vi "RTHost.vi"() -> ()   [LabVIEW 2013]
uses:
  <vilib>/Platform/TimedLoop/XDataNode/timing_clust.ctl
  <vilib>/Platform/TimedLoop/XDataNode/nitl_modes.ctl
  <vilib>/Platform/TimedLoop/XDataNode/wakeup.ctl
  <vilib>/FPGAPlugInAG/sbRIO-9632/niLvFpga_Open_sbRIO-9632.vi
  <vilib>/Utility/error.llb/Error Cluster From Error Code.vi
  <vilib>/rvi/errors/niLvFpgaAdjustHostInterfaceError.vi
  <vilib>/FPGAPlugInAG/sbRIO-9632/niLvFpga_Close_sbRIO-9632.vi
  <vilib>/rvi/interface/nirviOpenFPGA/nirviOpenFPGA.xnode
  FPGA Bitfiles/VMS15_FPGATarget_RTHost_BpHY6it1LyU.lvbitx
  <vilib>/rvi/interface/nirviReadWriteControl/nirviReadWriteControl.xnode
  <vilib>/Platform/TimedLoop/XDataNode/XDataNode.xnode
  <vilib>/rvi/interface/nirviCloseFPGA/nirviCloseFPGA.xnode
  NiFpgaLv.dll
  <vilib>/Platform/TimedLoop/XDataNode/XDNodeRunTimeDep.lvlib
panel:
  out "电池过温":bool
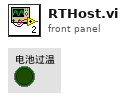
[diagram p1: front panel]
types:
  T1 = typedef "XDNodeRunTimeDep.lvlib/timing_clust.ctl" = cluster{"Expected End [f-1]":u64, "Actual End [f-1]":u64, "Finished Late? [f-1]":bool, "Expected End [i-1]":u64, "Actual End [i-1]":u64, "Finished Late? [i-1]":bool, "Expected Start [i]":u64, "Actual Start [i]":u64, "Expected Start [f]":u64, "Actual Start [f]":u64, "Source Name":string, "Structure Name":string, "Period":i64, "Deadline":i64, "Offset":i64, "Start":i64, "Priority":i32, "Timeout":i32, "Mode":T2, "Wakeup Reason":T3, "Error":errorcluster, "Source Type":string, "Secondary Source Type":string, "Global End Time":u64, "Global Start Time":u64, "Frame Duration":u64, "Iteration Duration":u64, "Assigned CPU":i32, "I/O Scan Engine Mode":u32}
  T2 = typedef "XDNodeRunTimeDep.lvlib/nitl_modes.ctl" = enum32{"No Change", "Process missed periods, maintain original phase", "Discard missed periods, maintain original phase", "Process missed periods, ignore original phase", "Discard missed periods, ignore original phase"}
  T3 = typedef "XDNodeRunTimeDep.lvlib/wakeup.ctl" = enum32{"Normal", "Aborted", "Asynchronous wakeup", "Timing source error", "Timed loop error", "Timeout"}
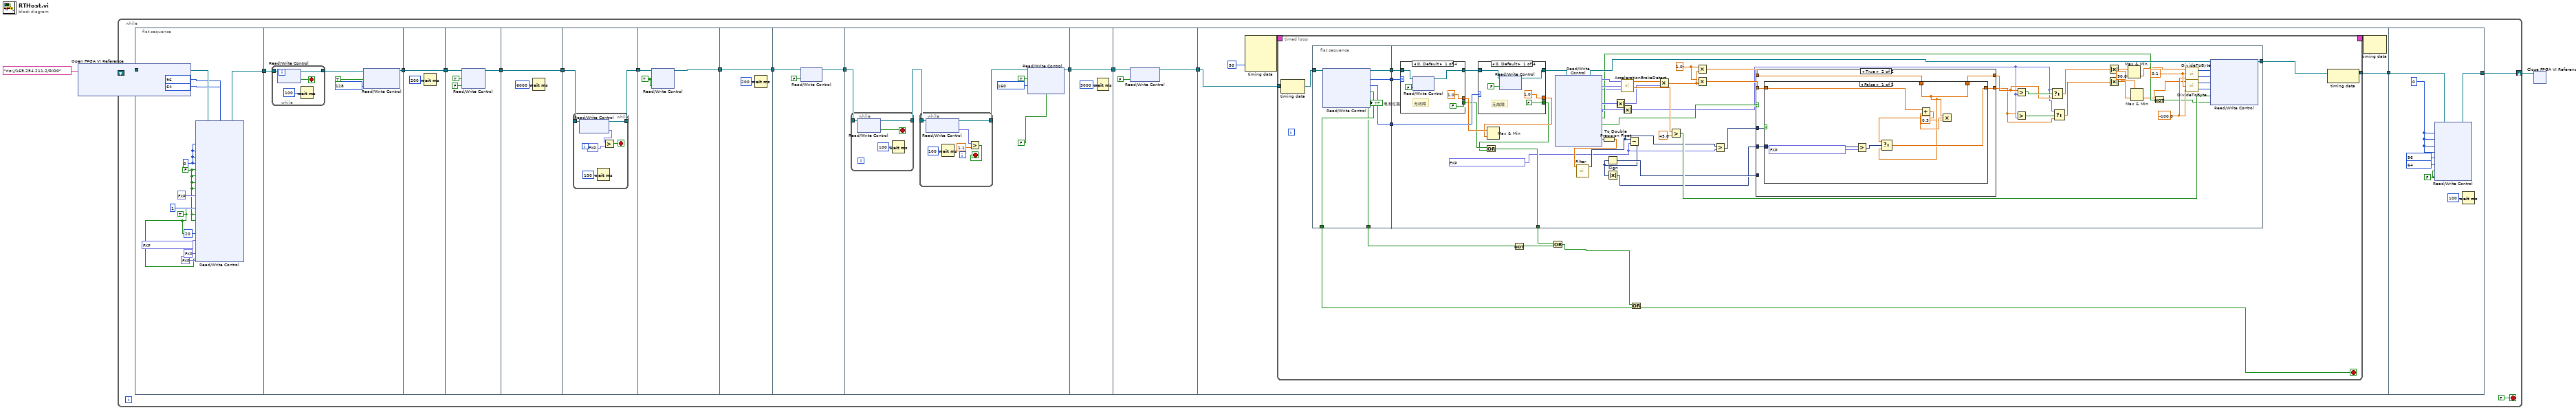
[diagram p0: block diagram]
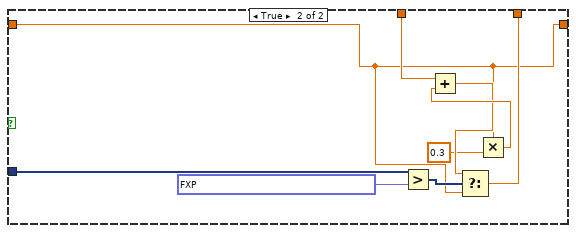
[diagram p3: hidden frame]
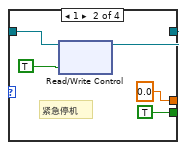
[diagram p4: hidden frame]
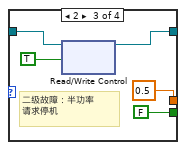
[diagram p5: hidden frame]
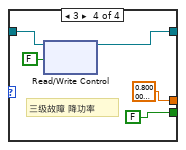
[diagram p6: hidden frame]
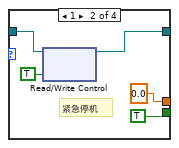
[diagram p7: hidden frame]
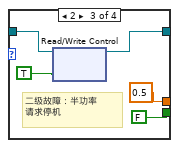
[diagram p8: hidden frame]
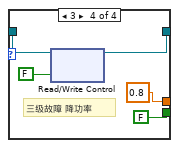
[diagram p9: hidden frame]
diagram:
  n1 = xnode "Open FPGA VI Reference"("resource name"=tag "rio://169.254.211.2/RIO0") -> ("FPGA VI Reference Out"=w1:refnum<k20>)  [unwired: 1 in, 1 out]
  n2 = while {
    shift-right: [w4] -> w2
    shift-left: w1 -> [w19]
    stop <- FALSE stop-if-true
    n3 = flat-sequence {
      tunnel: w19 -> [w29]
      tunnel: [w28] -> w18
      tunnel: w18 -> [w34]
      tunnel: [w33] -> w17
      tunnel: w17 -> [w43]
      tunnel: [w43] -> w16
      tunnel: w16 -> [w46]
      tunnel: [w45] -> w15
      tunnel: w15 -> [w49]
      tunnel: [w49] -> w10
      tunnel: [w51] -> w14
      tunnel: w10 -> [w50]
      tunnel: w14 -> [w60]
      tunnel: [w59] -> w7
      tunnel: w7 -> [w62]
      tunnel: [w62] -> w6
      tunnel: w6 -> [w65]
      tunnel: [w64] -> w5
      tunnel: w5 -> [w72]
      tunnel: [w67] -> w13
      tunnel: w13 -> [w84]
      tunnel: [w84] -> w9
      tunnel: [w86] -> w12
      tunnel: w9 -> [w87]
      tunnel: w12 -> [w90]
      tunnel: [w89] -> w11
      tunnel: w11 -> [w243]
      tunnel: [w238] -> w4
      frame #0 {
        w20 = TRUE ("AMS")
        w31 = u8 0 ("Byte 7")
        w21 = FALSE ("MotorAlarm?")
        n4 = xnode "Read/Write Control"("FPGA VI Reference In"=w29, "MCCmdByte"=u8 96, "BMCmdByte"=u8 64, "MC1TqSet_L"=w31, "MC1TqSet_H"=w31, "MC2TqSet_L"=w31, "MC2TqSet_H"=w31, "PREO"=w21, "AIRPO"=w21, "AIRNO"=w21, "BRAKELO"=w21, "开风扇温度值"=fxp<+,8,6> 60.0, "发送间隔(mSec)"=u8 1, "AMS"=w20, "BA"=w21, "MA"=w21, "接收窗口(mSec)"=u8 20, "Ready"=w20, "刹车标定上限"=fxp<+,32,16> 1.8000030517578125, "PowerPermitted"=fxp<+/-,64,32> 80.0, "开水泵温度值"=fxp<+/-,32,16> 60.0, "ErrorMonitoring?"=w20) -> ("FPGA VI Reference Out"=w28:refnum<k20>)  [unwired: 1 in, 1 out]
      }
      frame #1 {
        n5 = while {
          tunnel: w34 -> [w41]
          tunnel: [w40] -> w35
          stop <- w38 stop-if-true
          n6 = xnode "Read/Write Control"("FPGA VI Reference In"=w41) -> ("FPGA VI Reference Out"=w40:refnum<k20>, "Start？"=w38:bool)  [unwired: 1 in, 1 out]
          n7 = Wait (ms)(milliseconds to wait=u32 100) -> ()  [unwired: 1 out]
        }
        n8 = xnode "Read/Write Control"("FPGA VI Reference In"=w35, "PREO"=TRUE, "BMCmdByte"=u8 128) -> ("FPGA VI Reference Out"=w33:refnum<k20>)  [unwired: 1 in, 1 out]
      }
      frame #2 {
        n9 = Wait (ms)(milliseconds to wait=u32 200) -> ()  [unwired: 1 out]
      }
      frame #3 {
        n10 = xnode "Read/Write Control"("FPGA VI Reference In"=w46, "AIRNO"=TRUE, "Ready"=FALSE) -> ("FPGA VI Reference Out"=w45:refnum<k20>)  [unwired: 1 in, 1 out]
      }
      frame #4 {
        n11 = Wait (ms)(milliseconds to wait=u32 6000) -> ()  [unwired: 1 out]
      }
      frame #5 {
        n12 = while {
          tunnel: [w57] -> w51
          tunnel: w50 -> [w54]
          stop <- w52 stop-if-true
          n13 = xnode "Read/Write Control"("FPGA VI Reference In"=w54) -> ("FPGA VI Reference Out"=w57:refnum<k20>, "MC1VinIs"=w55:fxp<+/-,32,16>)  [unwired: 1 in, 1 out]
          n14 = Wait (ms)(milliseconds to wait=u32 100) -> ()  [unwired: 1 out]
          n15 = Greater?(x=w55, y=fxp<+,18,10> 480.0) -> (0:w52:bool)
        }
      }
      frame #6 {
        w58 = TRUE ("AIRPO")
        n16 = xnode "Read/Write Control"("FPGA VI Reference In"=w60, "AIRPO"=w58, "Ready"=w58) -> ("FPGA VI Reference Out"=w59:refnum<k20>)  [unwired: 1 in, 1 out]
      }
      frame #7 {
        n17 = Wait (ms)(milliseconds to wait=u32 200) -> ()  [unwired: 1 out]
      }
      frame #8 {
        n18 = xnode "Read/Write Control"("FPGA VI Reference In"=w65, "PREO"=FALSE) -> ("FPGA VI Reference Out"=w64:refnum<k20>)  [unwired: 1 in, 1 out]
      }
      frame #9 {
        n19 = while {
          tunnel: w72 -> [w76]
          tunnel: [w75] -> w71
          stop <- w73 stop-if-true
          n20 = xnode "Read/Write Control"("FPGA VI Reference In"=w76) -> ("FPGA VI Reference Out"=w75:refnum<k20>, "Start？"=w73:bool)  [unwired: 1 in, 1 out]
          n21 = Wait (ms)(milliseconds to wait=u16 100) -> ()  [unwired: 1 out]
        }
        n22 = while {
          tunnel: w71 -> [w80]
          tunnel: [w79] -> w70
          stop <- w77 stop-if-true
          n23 = xnode "Read/Write Control"("FPGA VI Reference In"=w80) -> ("FPGA VI Reference Out"=w79:refnum<k20>, "SIG_BRAKE"=w78:fxp<+/-,30,9>)  [unwired: 1 in, 1 out]
          n24 = Wait (ms)(milliseconds to wait=u16 100) -> ()  [unwired: 1 out]
          n25 = Greater?(x=w78, y=1.1) -> (0:w77:bool)
        }
        n26 = xnode "Read/Write Control"("FPGA VI Reference In"=w70, "BUZZERO"=TRUE, "MCCmdByte"=u8 160 ("CAN 4"), "Ready"=FALSE) -> ("FPGA VI Reference Out"=w67:refnum<k20>)  [unwired: 1 in, 1 out]
      }
      frame #10 {
        n27 = Wait (ms)(milliseconds to wait=u32 3000) -> ()  [unwired: 1 out]
      }
      frame #11 {
        n28 = xnode "Read/Write Control"("FPGA VI Reference In"=w87, "BUZZERO"=FALSE) -> ("FPGA VI Reference Out"=w86:refnum<k20>)  [unwired: 1 in, 1 out]
      }
      frame #12 {
        n29 = node-c288(i64 50 ("Period")) -> (w92:T1)  [unwired: 3 in]
        n30 = timed-loop {
          timing: w92 -> [_]
          timing-out: [_] -> w91
          tunnel: w90 -> [w102]
          tunnel: [w103] -> w89
          stop <- w94 stop-if-true
          n31 = node-c288() -> ()  [unwired: 1 in, 1 out]
          n32 = flat-sequence {
            tunnel: w102 -> [w107]
            tunnel: [w106] -> w98
            tunnel: [w110] -> w101
            tunnel: [w109] -> w100
            tunnel: [w108] -> w99
            tunnel: [w105] -> w96
            tunnel: w101 -> [w165]
            tunnel: w100 -> [w163]
            tunnel: w99 -> [w152]
            tunnel: [w153] -> w103
            tunnel: [w140] -> w97
            frame #0 {
              n33 = xnode "Read/Write Control"("FPGA VI Reference In"=w107) -> ("FPGA VI Reference Out"=w108:refnum<k20>, "BatteryErrorRank"=w110:u8, "MotorErrorRank"=w109:u8, "Stop？"=w106:bool, "SHTD"=w105:bool, "电池过温"=→"电池过温":bool)  [unwired: 1 in, 1 out]
            }
            frame #1 {
              w117 = 1.0 ("x")
              w134 = 90.0 ("y")
              w119 = fxp<+,29,3> 0.414000004529953 ("x")
              w156 = -100.0 ("Offset")
              w155 = 0.1 ("Resolution")
              n34 = case shown="0, Default" w165 {
                tunnel: [1.0 0.0 sgl 0.5 0.8] -> w162
                tunnel: [FALSE TRUE FALSE FALSE] -> w160
                tunnel: [w214 w218 w222 w227] -> w164
                tunnel: w152 -> [w213 w219 w223 w228]
                frame 0, Default {
                  # "无故障"
                  n35 = xnode "Read/Write Control"("FPGA VI Reference In"=w213, "BA"=FALSE ("Alarm")) -> ("FPGA VI Reference Out"=w214:refnum<k20>)  [unwired: 1 in, 1 out]
                }
                frame 1 {
                  # "紧急停机"
                  n36 = xnode "Read/Write Control"("FPGA VI Reference In"=w219, "BA"=TRUE) -> ("FPGA VI Reference Out"=w218:refnum<k20>)  [unwired: 1 in, 1 out]
                }
                frame 2 {
                  # "二级故障：半功率\n请求停机"
                  n37 = xnode "Read/Write Control"("FPGA VI Reference In"=w223, "BA"=TRUE ("Alarm")) -> ("FPGA VI Reference Out"=w222:refnum<k20>)  [unwired: 1 in, 1 out]
                }
                frame 3 {
                  # "三级故障 降功率"
                  n38 = xnode "Read/Write Control"("FPGA VI Reference In"=w228, "BA"=FALSE ("Alarm")) -> ("FPGA VI Reference Out"=w227:refnum<k20>)  [unwired: 1 in, 1 out]
                }
              }
              n39 = case shown="0, Default" w163 {
                tunnel: [1.0 0.0 sgl 0.5 sgl 0.8] -> w161
                tunnel: [w195 w201 w205 w209] -> w158
                tunnel: [FALSE TRUE FALSE FALSE] -> w159
                tunnel: w164 -> [w192 w199 w202 w207]
                frame 0, Default {
                  # "无故障"
                  n40 = xnode "Read/Write Control"("FPGA VI Reference In"=w192, "MA"=FALSE ("Alarm")) -> ("FPGA VI Reference Out"=w195:refnum<k20>)  [unwired: 1 in, 1 out]
                }
                frame 1 {
                  # "紧急停机"
                  n41 = xnode "Read/Write Control"("FPGA VI Reference In"=w199, "MA"=TRUE) -> ("FPGA VI Reference Out"=w201:refnum<k20>)  [unwired: 1 in, 1 out]
                }
                frame 2 {
                  # "二级故障：半功率\n请求停机"
                  n42 = xnode "Read/Write Control"("FPGA VI Reference In"=w202, "MA"=TRUE ("Alarm")) -> ("FPGA VI Reference Out"=w205:refnum<k20>)  [unwired: 1 in, 1 out]
                }
                frame 3 {
                  # "三级故障 降功率"
                  n43 = xnode "Read/Write Control"("FPGA VI Reference In"=w207, "MA"=FALSE ("Alarm")) -> ("FPGA VI Reference Out"=w209:refnum<k20>)  [unwired: 1 in, 1 out]
                }
              }
              n44 = Or(x=w160, y=w159) -> (x .or. y?=w140:bool)
              n45 = Max & Min(x=w162, y=w161) -> ()  [unwired: 2 out]
              n46 = xnode "Read/Write Control"("FPGA VI Reference In"=w158) -> ("FPGA VI Reference Out"=w151:refnum<k20>, "SIG_ACC1"=w148:fxp<+/-,30,9>, "SIG_ACC2"=w147:fxp<+/-,30,9>, "SIG_BRAKE"=w132:fxp<+/-,30,9>, "PowerLimited"=w149:fxp<+/-,16,6>, "TorquePermitted"=w145:fxp<+/-,64,40>, "SWT3?"=w144:bool, "SWT4?"=w139:bool, "LinRR"=w122:fxp<+/-,32,16>)  [unwired: 1 in, 3 out]
              n47 = To Double Precision Float(number=w122) -> (double precision float=w121:dbl)
              n48 = call "Filter"("Signal"=w121) -> ("Filtered Signal"=w120:dynamicdata)  [unwired: 9 in, 1 out]
              n49 = Absolute Value(x=w149) -> (abs(x)=w131:fxp<+,16,6>)
              n50 = call "AccelerationBrakeDetect.vi"("油门1输入"=w148, "油门2输入"=w147, "刹车输入"=w132) -> ("油门1"=w150:dbl, "刹车"=w154:dbl)  [unwired: 3 out]
              n51 = Absolute Value(x=w145) -> (abs(x)=w125:fxp<+,64,40>)
              n52 = Subtract(x=w120, y=w119) -> (x-y=w137:dynamicdata)
              n53 = Sign(1:w137) -> (0:w141:dynamicdata)
              n54 = Absolute Value(x=w137) -> (abs(x)=w138:dynamicdata)
              n55 = Multiply(x=w150, y=w131) -> (x*y=w123:dbl)
              n56 = Greater?(x=w154, y=45.0) -> (0:w146:bool)
              n57 = Multiply(x=w117, y=w123) -> (x*y=w143:dbl)
              n58 = Multiply(x=w117, y=w123) -> (x*y=w142:dbl)
              n59 = Greater?(x=w120, y=w119) -> (0:w118:dynamicdata)
              n60 = case shown="True" w139 {
                tunnel: w143 -> [w167 w173]
                tunnel: w142 -> [w166 w172]
                tunnel: [w167 w171] -> w129
                tunnel: [w166 w170] -> w124
                tunnel: w141 -> [_ _]
                tunnel: w138 -> [_ w169]
                tunnel: w118 -> [_ w168]
                frame False {
                }
                frame True {
                  n61 = case shown="False" w168 {
                    tunnel: w173 -> [w175 w191]
                    tunnel: w172 -> [w182 w184]
                    tunnel: [w175 w185] -> w171
                    tunnel: [w176 w184] -> w170
                    tunnel: w169 -> [w180 w189]
                    frame False {
                      n62 = Greater?(x=w180, y=fxp<+,29,3> 0.09999999403953552) -> (0:w178:dynamicdata)
                      n63 = Multiply(x=w175, y=0.3) -> (x*y=w181:dbl)
                      n64 = Add(x=w182, y=w181) -> (x+y=w177:dbl)
                      n65 = Select(t=w177, s=w178, f=w175) -> (s? t:f=w176:dbl)
                    }
                    frame True {
                      n66 = Greater?(x=w189, y=fxp<+,29,3> 0.2810000032186508) -> (0:w187:dynamicdata)
                      n67 = Multiply(x=w184, y=0.3) -> (x*y=w190:dbl)
                      n68 = Add(x=w191, y=w190) -> (x+y=w186:dbl)
                      n69 = Select(t=w186, s=w187, f=w184) -> (s? t:f=w185:dbl)
                    }
                  }
                }
              }
              n70 = Greater?(x=w129, y=w125) -> (0:w130:bool)
              n71 = Greater?(x=w124, y=w125) -> (0:w126:bool)
              n72 = Select(t=w125, s=w130, f=w129) -> (s? t:f=w128:dbl)
              n73 = Select(t=w125, s=w126, f=w124) -> (s? t:f=w127:dbl)
              n74 = Absolute Value(x=w128) -> (abs(x)=w135:dbl)
              n75 = Absolute Value(x=w127) -> (abs(x)=w136:dbl)
              n76 = Max & Min(x=w135, y=w134) -> (min(x,y)=w115:dbl)  [unwired: 1 out]
              n77 = Max & Min(x=w134, y=w136) -> (min(x,y)=w116:dbl)  [unwired: 1 out]
              n78 = Not(x=w144) -> (.not. x?=w133:bool)
              n79 = call "DivideToByte.vi"("Offset"=w156, "Resolution"=w155, "Value"=w115) -> ("HighByte"=w113:u8, "LowByte"=w114:u8)
              n80 = call "DivideToByte.vi"("Offset"=w156, "Resolution"=w155, "Value"=w116) -> ("HighByte"=w111:u8, "LowByte"=w112:u8)
              n81 = xnode "Read/Write Control"("FPGA VI Reference In"=w151, "MC1TqSet_L"=w114, "MC1TqSet_H"=w113, "MC2TqSet_L"=w112, "MC2TqSet_H"=w111, "BRAKELO"=w146, "ErrorMonitoring?"=w133) -> ("FPGA VI Reference Out"=w153:refnum<k20>)  [unwired: 1 in, 1 out]
            }
          }
          n82 = Not(x=w96) -> (.not. x?=w95:bool)
          n83 = Or(x=w97, y=w95) -> (x .or. y?=w93:bool)
          n84 = Or(x=w93, y=w98) -> (x .or. y?=w94:bool)
          n85 = node-c288() -> ()  [unwired: 1 in, 1 out]
        }
        n86 = node-c288(w91) -> ()  [unwired: 1 out]
      }
      frame #13 {
        w239 = FALSE ("AIRNO")
        w242 = u8 0 ("CAN 0")
        n87 = xnode "Read/Write Control"("FPGA VI Reference In"=w243, "MC1TqSet_L"=w242, "MC1TqSet_H"=w242, "MC2TqSet_L"=w242, "MC2TqSet_H"=w242, "MCCmdByte"=u8 96 ("CAN 5"), "BMCmdByte"=u8 64 ("CAN 4"), "AIRPO"=w239, "AIRNO"=w239) -> ("FPGA VI Reference Out"=w238:refnum<k20>)  [unwired: 1 in, 1 out]
        n88 = Wait (ms)(milliseconds to wait=u32 100) -> ()  [unwired: 1 out]
      }
    }
  }
  n89 = xnode "Close FPGA VI Reference"("FPGA VI Reference In"=w2) -> ()  [unwired: 1 in, 1 out]
